vi "Boolcvrt.vi"(6 "ORide":bool=TRUE, 8 "error in":errorcluster, 9 "Bool Refnum":refnum<vi>) -> (0 "error out":errorcluster, 1 "T/F":bool)   [LabVIEW 2018, in "PNA-X.lvlib"]
uses:
  PNA-X.lvlib
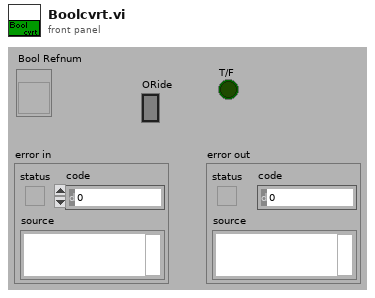
[diagram p1: front panel]
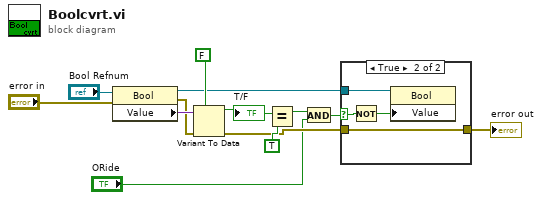
[diagram p0: block diagram]
diagram:
  n1 = property class="Bool"(reference="Bool Refnum", error in="error in") -> (reference out=w5:refnum<vi>, error out=w11:errorcluster, "Value"=w12:variant)
  n2 = Variant To Data(error in=w11, type=FALSE, Variant=w12) -> (data=w8:bool, error out=w6:errorcluster)
  "T/F" <- w8
  n3 = Equal?(x=w8, y=TRUE) -> (x = y?=w3:bool)
  n4 = And(x=w3, y="ORide") -> (x .and. y?=w2:bool)
  n5 = case shown="True" w2 {
    selector: w2 -> [_ w16]
    tunnel: w6 -> [w14 w17]
    tunnel: w5 -> [_ w18]
    tunnel: [w14 w17] -> w4
    frame False {
    }
    frame True {
      n6 = Not(x=w16) -> (.not. x?=w15:bool)
      n7 = property class="Bool"(reference=w18, "Value"=w15) -> ()  [unwired: 1 in, 2 out]
    }
  }
  "error out" <- w4
